vi "Get Chassis Information.vi"(8 "error in":errorcluster, 11 "Controller in":refnum<class "Controller.lvclass">) -> (0 "error out":errorcluster, 2 "Chassis Information":T3 {"Remote Chassis"."Modules"."Module Code" format="%.0x"; "Local Chassis"."Modules"."Module Code" format="%.0x"}, 3 "Controller out":refnum<class "Controller.lvclass">)   [LabVIEW 2015, in "SMI.lvlib" / "Chassis.lvclass"]
uses:
  Chassis.lvclass
  Controller/Controller.lvclass
  Controls/ChassisInformation.ctl
  Module/Controls/ModuleInformation.ctl
  Controller/Controller.lvclass/Controller.ctl
  Device/Device.lvclass/Device.ctl
  Chassis.lvclass/Chassis.ctl
  Controller/Accessor Methods/Read Local Chassis.vi
  Controller/Accessor Methods/Read Remote Chassis.vi
  Device/Accessor Methods/Read Vendor Name.vi
  Device/Accessor Methods/Read Product Name.vi
  Device/Accessor Methods/Read Product ID.vi
  Device/Accessor Methods/Read Serial Number.vi
  Module/Module.lvclass
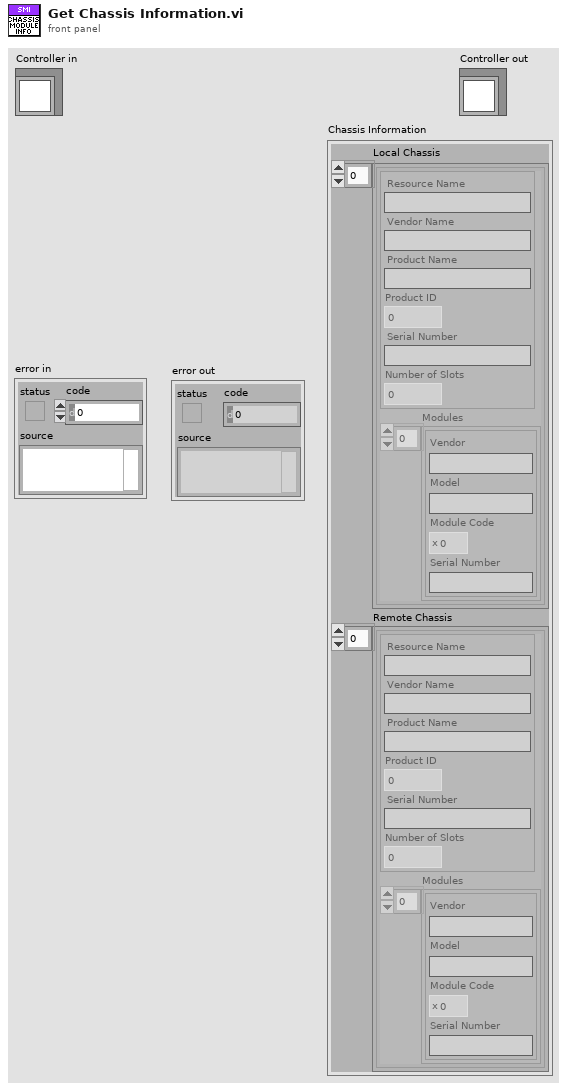
[diagram p1: front panel]
types:
  T1 = typedef "SMI.lvlib/Chassis.lvclass/ChassisInformation.ctl" = cluster{"Resource Name":string, "Vendor Name":string, "Product Name":string, "Product ID":u32, "Serial Number":string, "Number of Slots":i32}
  T2 = typedef "SMI.lvlib/Module.lvclass/ModuleInformation.ctl" = cluster{"Vendor":string, "Model":string, "Module Code":u32, "Serial Number":string}
  T3 = cluster{"Local Chassis":cluster{"Chassis":T1, "Modules":T2[]}[], "Remote Chassis":cluster{"Chassis":T1, "Modules":T2[]}[]}
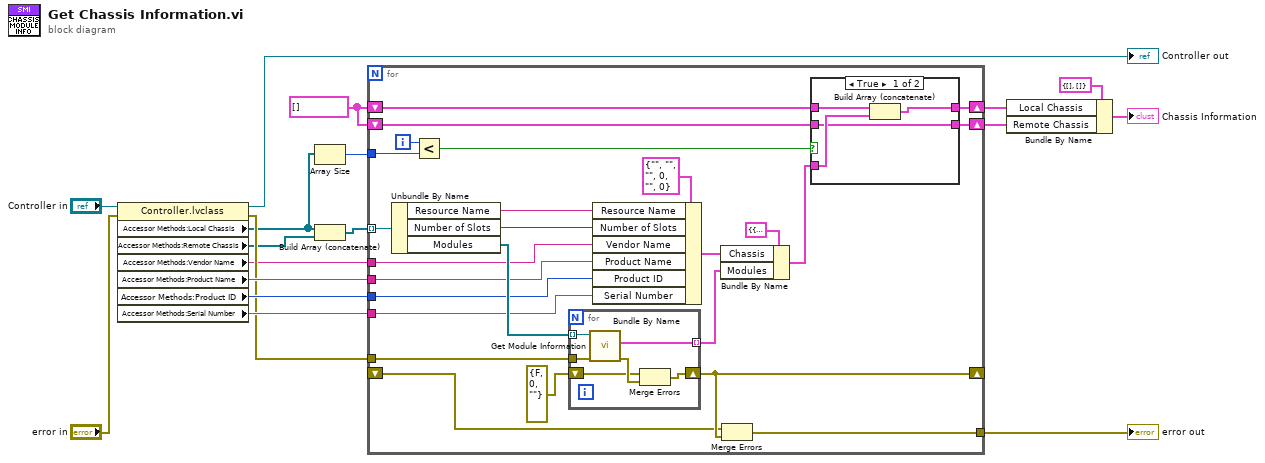
[diagram p0: block diagram]
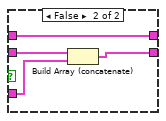
[diagram p2: hidden frame]
diagram:
  w2 = cluster{"Chassis":T1, "Modules":T2[]}[] []
  n1 = property class="Controller.lvclass"(reference="Controller in", error in="error in") -> (reference out=→"Controller out":refnum<class "Controller.lvclass">, error out=w13:errorcluster, "Accessor Methods:Local Chassis"=w10:refnum<class "Chassis.lvclass">[], "Accessor Methods:Remote Chassis"=w9:refnum<class "Chassis.lvclass">[], "Accessor Methods:Vendor Name"=w12:string, "Accessor Methods:Product Name"=w17:string, "Accessor Methods:Product ID"=w16:u32, "Accessor Methods:Serial Number"=w15:string)
  n2 = Array Size(array=w10) -> (size(s)=w5:i32)
  n3 = Build Array (concatenate)(w10, w9) -> (w6:refnum<class "Chassis.lvclass">[])
  n4 = for {
    tunnel: w6 -> [w43] mode=indexing
    tunnel: w13 -> [w40]
    tunnel: w12 -> [w36]
    tunnel: w17 -> [w35]
    tunnel: w16 -> [w34]
    tunnel: w15 -> [w33]
    tunnel: w5 -> [w28]
    shift-right: [w22] -> w4
    shift-left: w2 -> [w25]
    shift-right: [w23] -> w3
    shift-left: w2 -> [w26]
    shift-right: [w21] -> _
    shift-left: _ -> [w20]
    tunnel: [w19] -> w1
    i -> [w29]
    n5 = Unbundle By Name(w43) -> ("Resource Name"=w38:string, "Number of Slots"=w37:i32, "Modules"=w41:refnum<class "Module.lvclass">[])
    n6 = Less?(x=w29, y=w28) -> (x < y?=w27:bool)
    n7 = for {
      tunnel: w41 -> [w57] mode=indexing
      tunnel: [w56] -> w30 mode=indexing
      shift-right: [w52] -> w21
      shift-left: errorcluster {"status"=FALSE, "code"=0, "source"=""} ("error IO") -> [w53]
      tunnel: w40 -> [w55]
      n8 = call "Get Module Information.vi"("error in"=w55, "Module in"=w57) -> ("error out"=w54:errorcluster, "Module Information"=w56:T2)  [unwired: 7 in, 1 out]
      n9 = Merge Errors(w53, w54) -> (w52:errorcluster)
    }
    n10 = Bundle By Name(cluster=T1 {"Resource Name"="", "Vendor Name"="", "Product Name"="", "Product ID"=0, "Serial Number"="", "Number of Slots"=0} ("Chassis Information"), "Resource Name"=w38, "Number of Slots"=w37, "Vendor Name"=w36, "Product Name"=w35, "Product ID"=w34, "Serial Number"=w33) -> (w31:T1)
    n11 = Bundle By Name(cluster=cluster{"Chassis":T1, "Modules":T2[]} {"Chassis"={"Resource Name"="", "Vendor Name"="", "Product Name"="", "Product ID"=0, "Serial Number"="", "Number of Slots"=0}, "Modules"=[]} ("Chassis Information"), "Chassis"=w31, "Modules"=w30) -> (w24:cluster{"Chassis":T1, "Modules":T2[]})
    n12 = Merge Errors(w20, w21) -> (w19:errorcluster)
    n13 = case shown="True" w27 {
      tunnel: w26 -> [w47 w48]
      tunnel: w25 -> [w44 w49]
      tunnel: w24 -> [w45 w51]
      tunnel: [w46 w48] -> w23
      tunnel: [w44 w50] -> w22
      frame True {
        n14 = Build Array (concatenate)(w47, w45) -> (w46:cluster{"Chassis":T1, "Modules":T2[]}[])
      }
      frame False {
        n15 = Build Array (concatenate)(w49, w51) -> (w50:cluster{"Chassis":T1, "Modules":T2[]}[])
      }
    }
  }
  "error out" <- w1
  n16 = Bundle By Name(cluster=T3 {"Local Chassis"=[], "Remote Chassis"=[]} ("Chassis Information"), "Local Chassis"=w3, "Remote Chassis"=w4) -> (→"Chassis Information":T3)
